vi "2-complement convert.vi"(9 "2-complement input":u32=92 format="%.0b", 11 "Numer of bit":i32=16) -> (2 "2-complement value":i32)   [LabVIEW 2010]
doc: "Converts a number represented in two's complement form in the corresponding signed value"
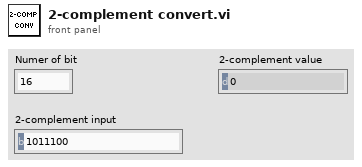
[diagram p1: front panel]
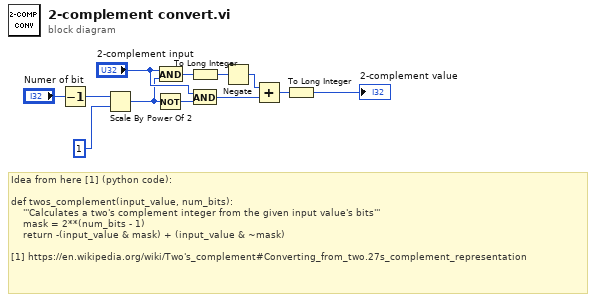
[diagram p0: block diagram]
diagram:
  # "Idea from here [1] (python code):\n\ndef twos_complement(input_value, num_bits):\n    '''Calculates a two's complement integer from the given input value's bits'''\n    mask = 2**(num_bits - 1)\n    return -(input_value & mask) + (input_value & ~mask)\n\n[1] https://en.wikipedia.org/wiki/Two's_complement#Converting_from_two.27s_complement_representation"
  n1 = Decrement(x="Numer of bit") -> (x-1=w5:i32)
  n2 = Scale By Power Of 2(n=w5, x=u32 1) -> (x*2^n=w3:u32)
  n3 = Not(x=w3) -> (.not. x?=w10:u32)
  n4 = And(x="2-complement input", y=w3) -> (x .and. y?=w7:u32)
  n5 = To Long Integer(number=w7) -> (32bit integer=w6:i32)
  n6 = And(x="2-complement input", y=w10) -> (x .and. y?=w9:u32)
  n7 = Negate(x=w6) -> (-x=w12:i32)
  n8 = Add(x=w12, y=w9) -> (x+y=w8:u32)
  n9 = To Long Integer(number=w8) -> (32bit integer=→"2-complement value":i32)
